vi "Read SubPanel Ref.vi"(8 "error in (no error)":errorcluster, 11 "Instrument Finder in":refnum<class "Instrument Finder.lvclass">) -> (0 "error out":errorcluster, 2 "SubPanel Ref":refnum<vi>, 3 "Instrument Finder out":refnum<class "Instrument Finder.lvclass">)   [LabVIEW 2014]
uses:
  Instrument Finder.lvclass
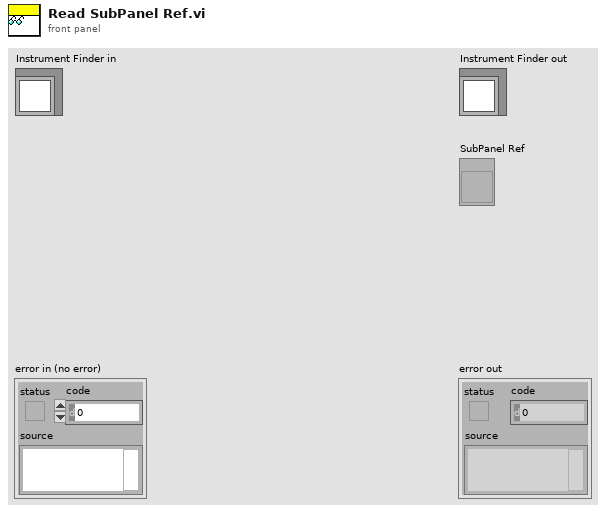
[diagram p1: front panel]
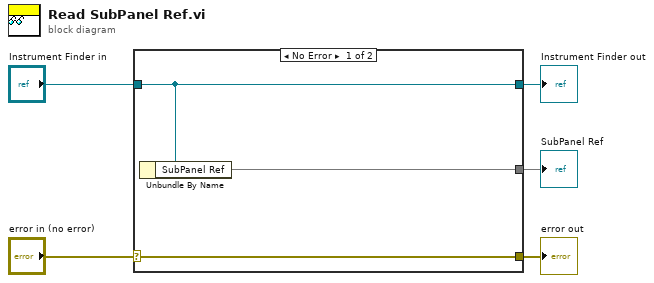
[diagram p0: block diagram]
diagram:
  n1 = case shown="No Error" "error in (no error)" {
    selector: "error in (no error)" -> [w8 w9]
    tunnel: [w8 w9] -> w4
    tunnel: [w7 w10] -> w2
    tunnel: "Instrument Finder in" -> [w7 w10]
    tunnel: [w6 _] -> w1
    frame No Error {
      n2 = Unbundle By Name(w7) -> ("SubPanel Ref"=w6)
    }
    frame Error {
    }
  }
  "error out" <- w4
  "Instrument Finder out" <- w2
  "SubPanel Ref" <- w1
